vi "chainCommands.vi"(9 "Command":string, 11 "String in":string) -> (3 "String 2":string)   [LabVIEW 2012]
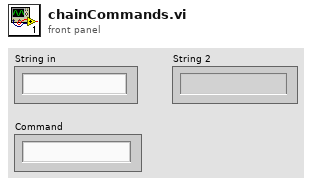
[diagram p1: front panel]
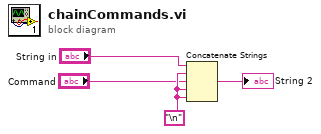
[diagram p0: block diagram]
diagram:
  w4 = "\n"
  n1 = Concatenate Strings("String in", w4, "Command", w4, w4) -> (→"String 2":string)
